vi "Set ByVal.vi"(8 "error in (no error)":errorcluster, 10 "Int":i32, 11 "Numeric in":refnum<class "Numeric Test Object.lvclass">) -> (0 "error out":errorcluster, 3 "Numeric out":refnum<class "Numeric Test Object.lvclass">)   [LabVIEW 2009, in "Numeric Test Object.lvclass"]
uses:
  Numeric Test Object.lvclass
  Numeric Test Object.lvclass/Numeric Test Object.ctl
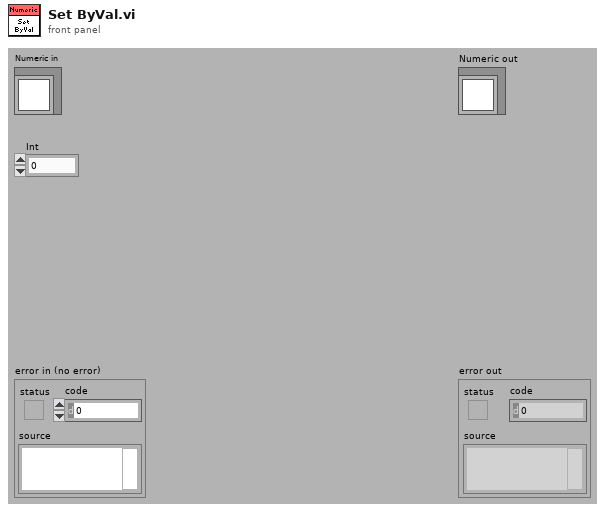
[diagram p1: front panel]
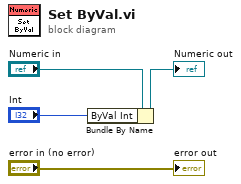
[diagram p0: block diagram]
diagram:
  n1 = Bundle By Name(cluster="Numeric in", "ByVal Int"="Int") -> (→"Numeric out":refnum<class "Numeric Test Object.lvclass">)
  "error out" <- "error in (no error)"
